vi "libera.vi"() -> ()   [LabVIEW 2012]
uses:
  chaos-common-crest/LabVIEW/LV14/chaosui-crest/chaosui-crest.lvlib
  chaos-common-crest/LabVIEW/LV14/chaosui-crest/VIs/ChaosDevState.ctl
  <vilib>/Utility/file.llb/Write To Spreadsheet File (I64).vi
  libera_env.ctl
panel:
  in  "[MT]:YYYYMMDDhhmm.ss":string
  in  "value":string
  in  "Set Environment":T1
  out "DD2":cluster{"VA":i32, "VB":i32, "VC":i32, "VD":i32}(graph)
  out "SA":cluster{"VA":i32, "VB":i32, "VC":i32, "VD":i32}(graph)
  out "DD":cluster{i32[], i32[]}[](graph)
  in  "DataFile":path
  out "libera_error":i32
  out "STATUS":string
  out "SA_OUT":T2(array[cluster])
  out "ADC_CW":T3(array[cluster])
  out "AVG_OUT":cluster{"AVG":i32}[](array[cluster])
  out "ADC_SP":T4(array[cluster])
  in  "AVG":bool=TRUE
  in  "STATE":bool=TRUE
  in  "stop":bool
  in  "loops":i32=10
  in  "DECIMATED":bool
  out "DD_OUT":T5(array[cluster])
  in  "refresh (ms)":u32=200
  out "samples":i32
  out "mode":i32
  out "Device State":T6
  out "nok":i32
  out "dev_error":bool
  out "acquisitions":u64
  out "timestamp":u64
  in  "Samples":u32=10
  in  "TRIGGERED":bool
  in  "ADC CW":bool
  in  "ADC SP":bool
  in  "SA":bool
  in  "DD":bool
  in  "!CHAOS URL":string="chaost-webui1.chaos.lnf.infn.it:8081"
  in  "LiberaID":string="LIBERA02/LIBERA_ACQUIRE0"
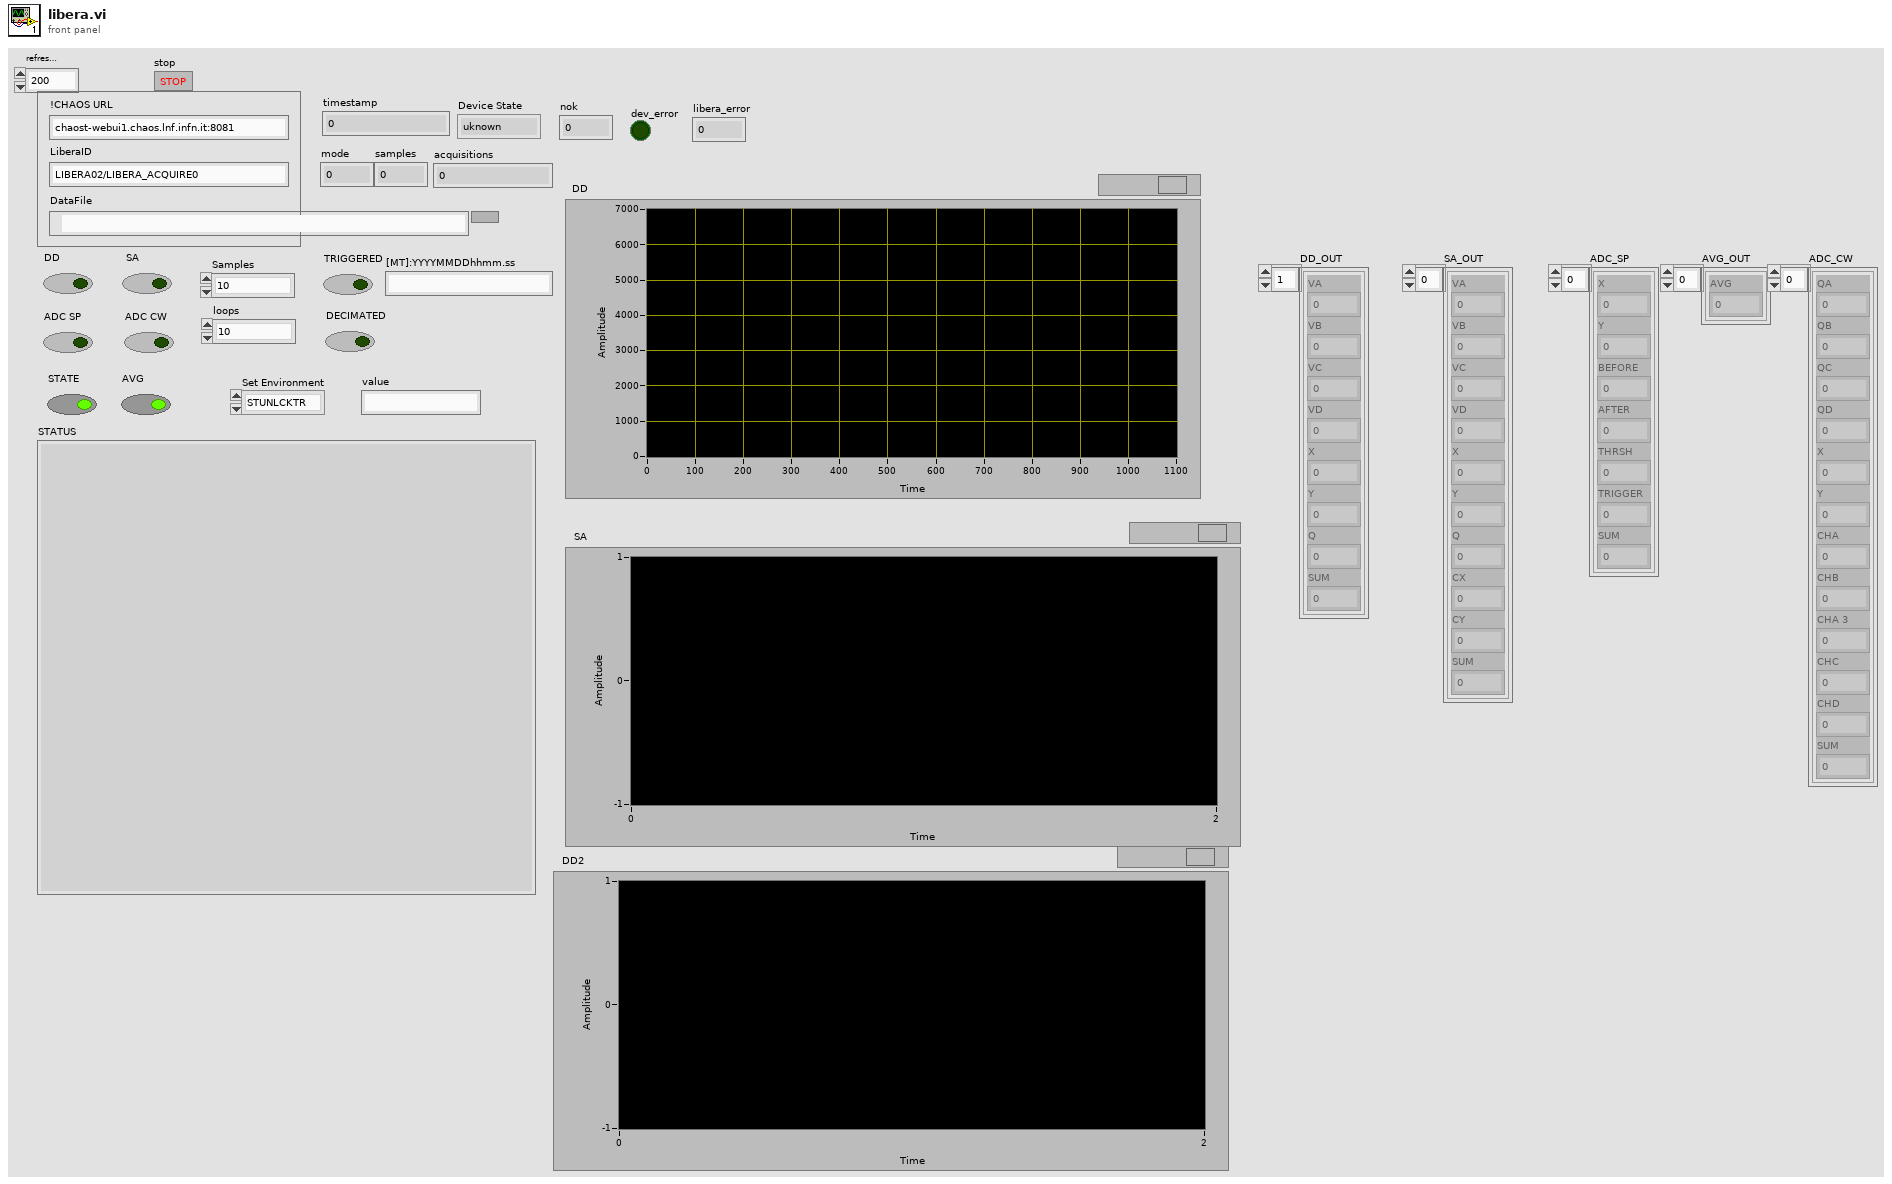
[diagram p1: front panel]
types:
  T1 = typedef "libera_env.ctl" = enum16{"STUNLCKTR", "MTSYNCIN", "MTUNLCKTR", "MTNCOSHFT", "MTVCXOFFS", "POLYPHASE_FIR", "NOTCH2", "NOTCH1", "DDC_MAFDELAY", "DDC_MAFLENGTH", "SWDELAY", "EXTSWITCH", "TRIGDELAY", "PMDEC", "PMOFFSET", "ILKSTATUS", "ILK", "DSC", "AGC", "GAIN", "SWITCH", "QOFFSET", "YOFFSET", "XOFFSET", "KY", "KX"}
  T2 = cluster{"VA":i32, "VB":i32, "VC":i32, "VD":i32, "X":i32, "Y ":i32, "Q":i32, "CX":i32, "CY":i32, "SUM":i32}[]
  T3 = cluster{"QA":i32, "QB":i32, "QC":i32, "QD":i32, "X":i32, "Y":i32, "CHA":i32, "CHB":i32, "CHA 3":i32, "CHC":i32, "CHD":i32, "SUM":i32}[]
  T4 = cluster{"X":i32, "Y":i32, "BEFORE":i32, "AFTER":i32, "THRSH":i32, "TRIGGER":i32, "SUM":i32}[]
  T5 = cluster{"VA":i32, "VB":i32, "VC":i32, "VD":i32, "X":i32, "Y ":i32, "Q":i32, "SUM":i32}[]
  T6 = typedef "ChaosDevState.ctl" = enum16{"uknown", "stop", "init", "deinit", "start"}
  T7 = typedef "LabVIEWHTTPClient.lvlib/ClientHandle.ctl" = refnum<k1>
  T8 = cluster{"client handle out":T7, "chaoswanurl":string}
  T9 = enum16{"setEnv", "stopAcquire", "setTime", "acquireAVG", "acquireADCSP", "acquireADCCW", "acquireStream", "acquireDD"}
  T10 = cluster{"VA":i32, "VB":i32, "VC":i32, "VD":i32, "X":i32, "Y ":i32, "Q":i32, "CX":i32, "CY":i32, "SUM":i32}
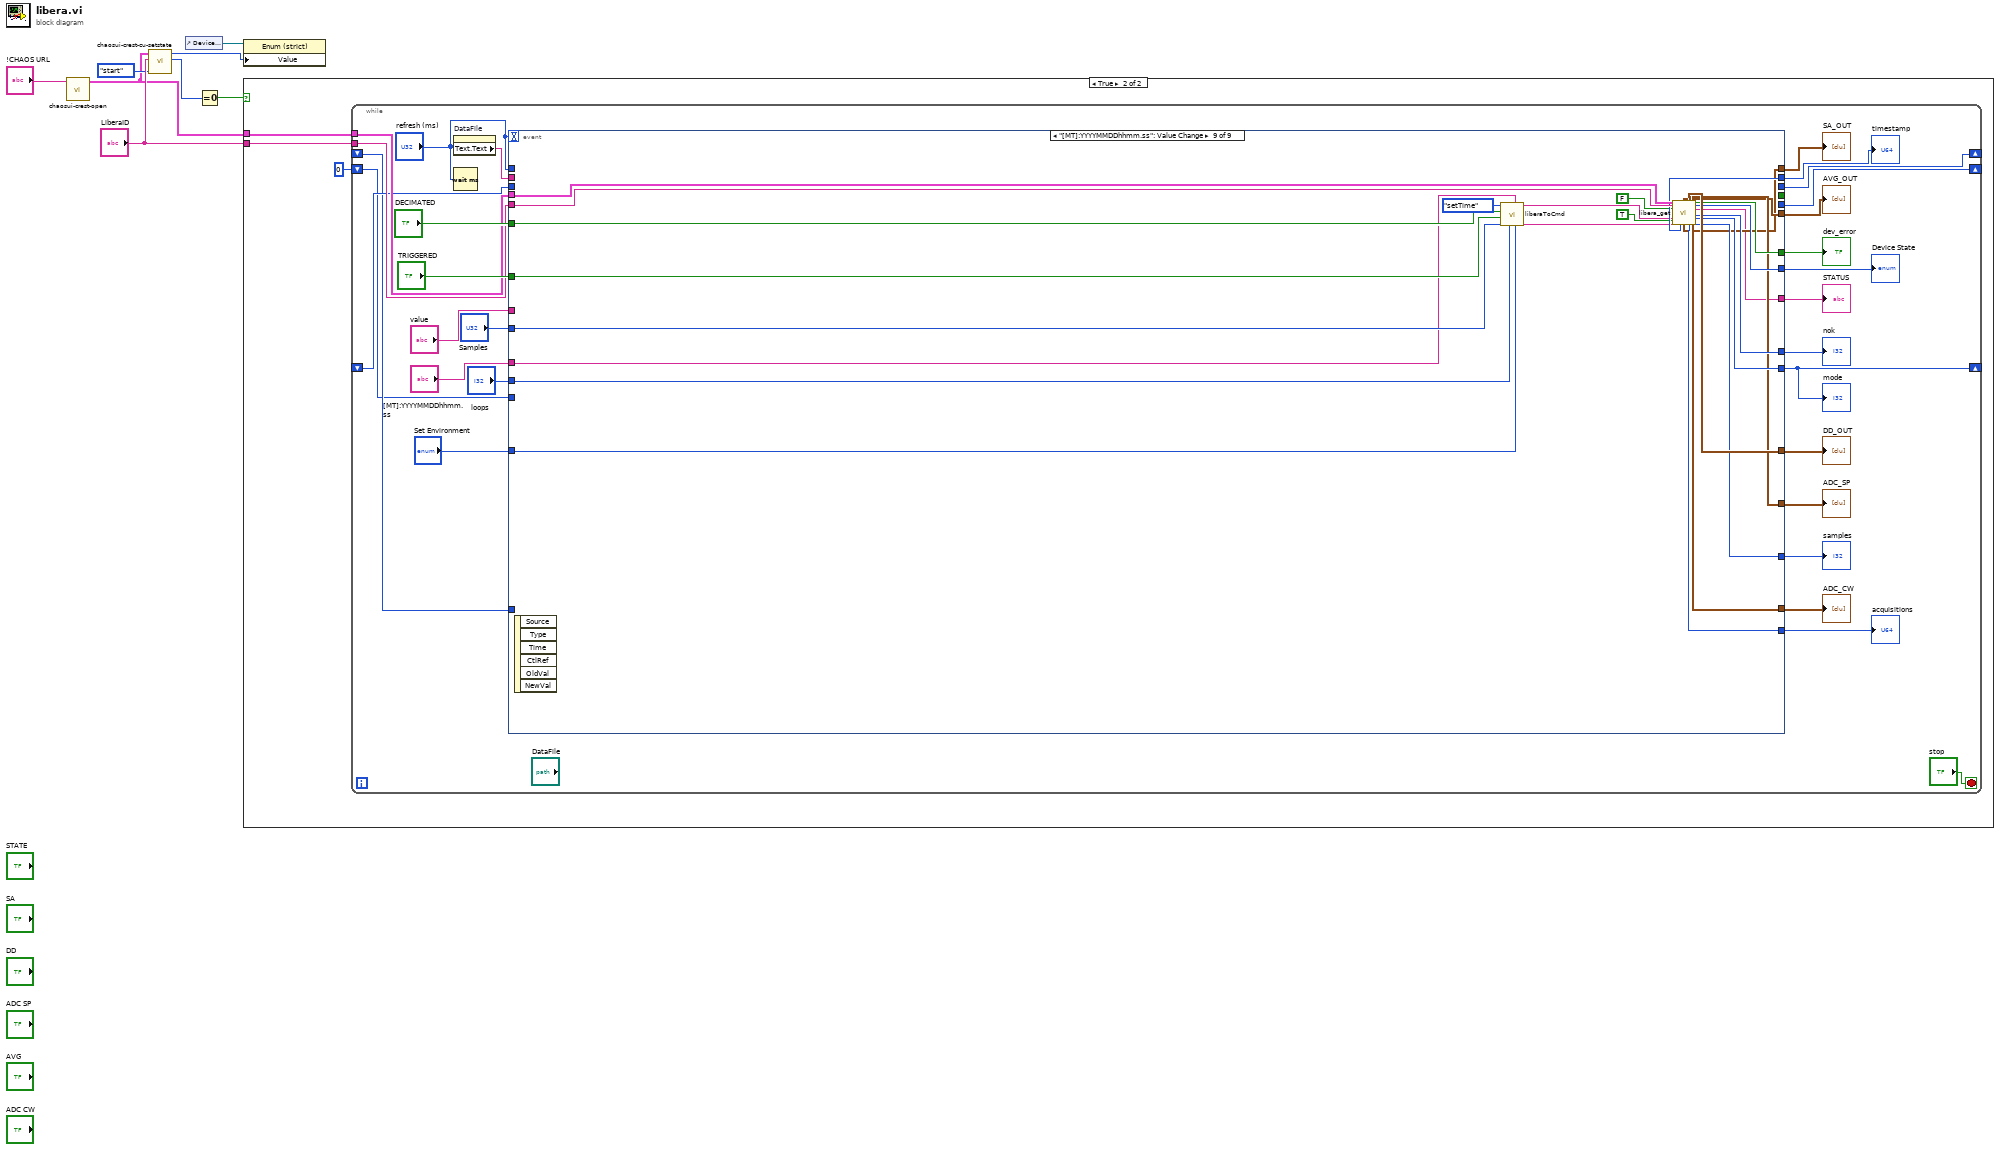
[diagram p0: block diagram]
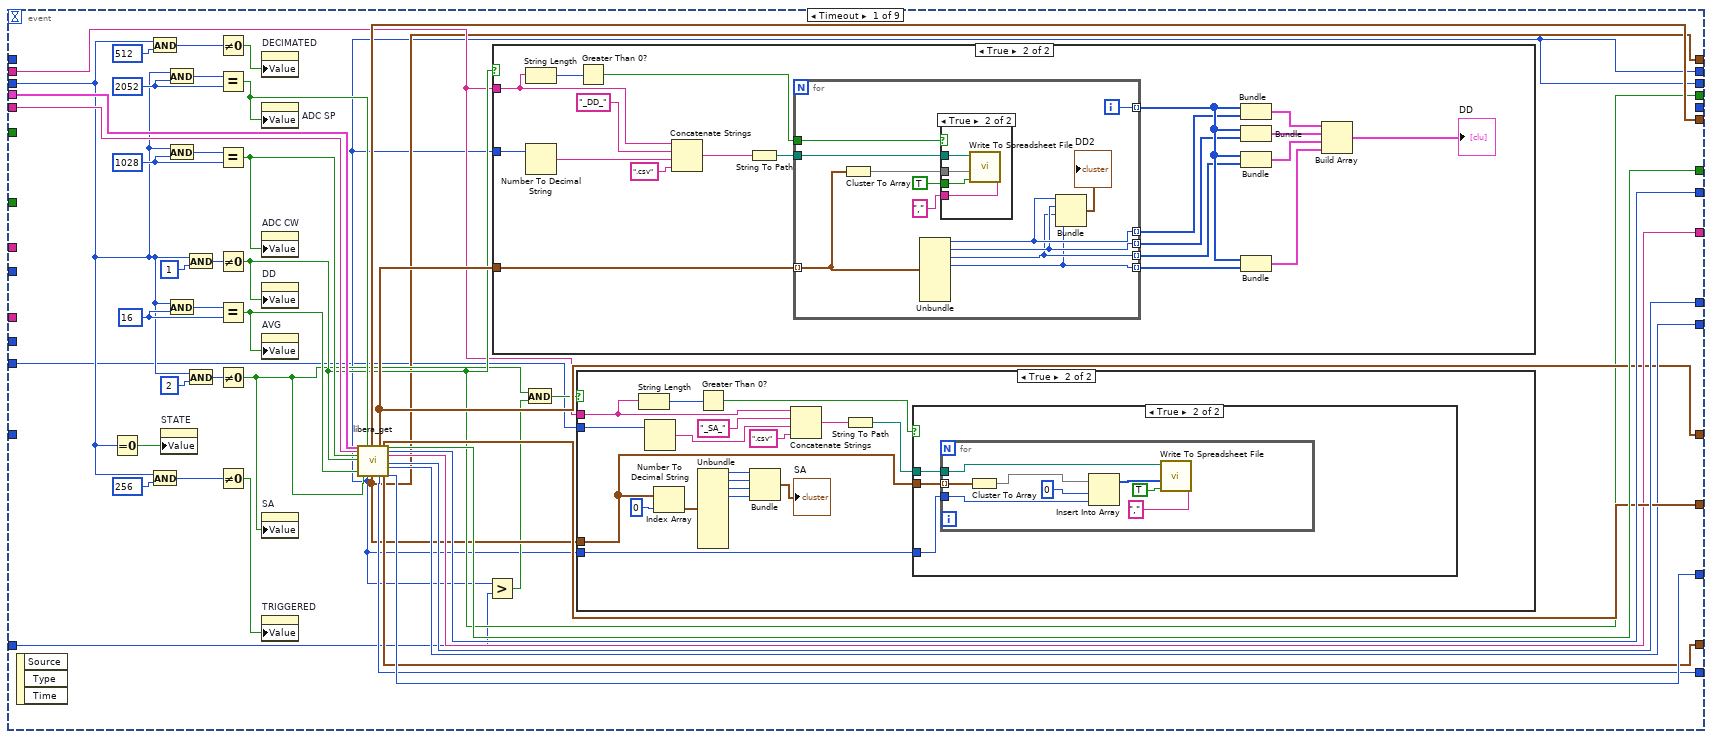
[diagram p3: hidden frame]
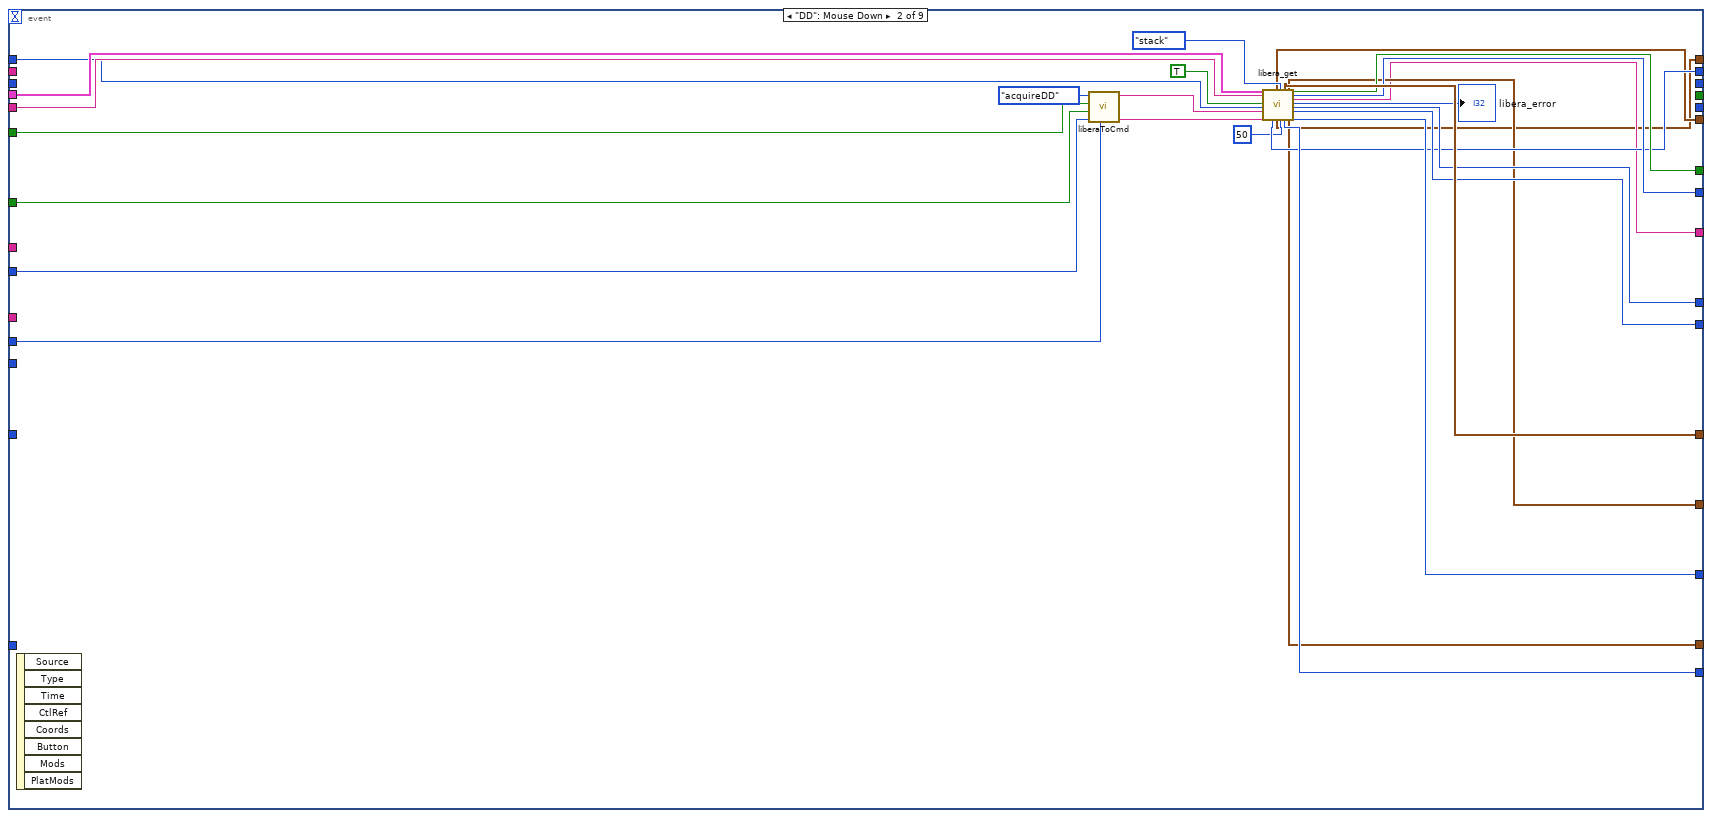
[diagram p8: hidden frame]
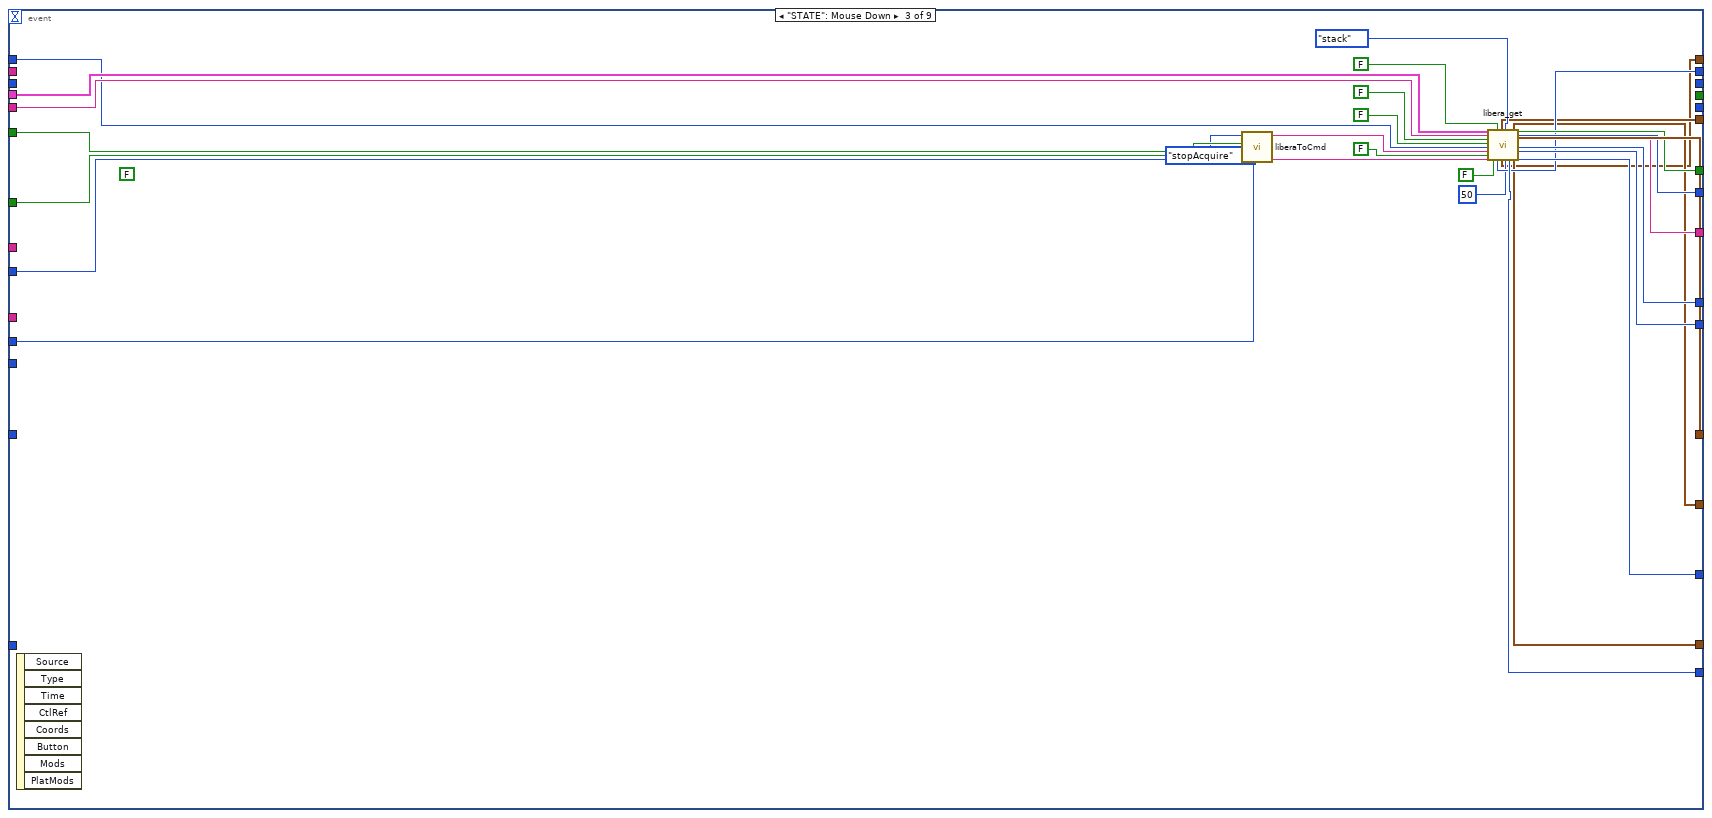
[diagram p9: hidden frame]
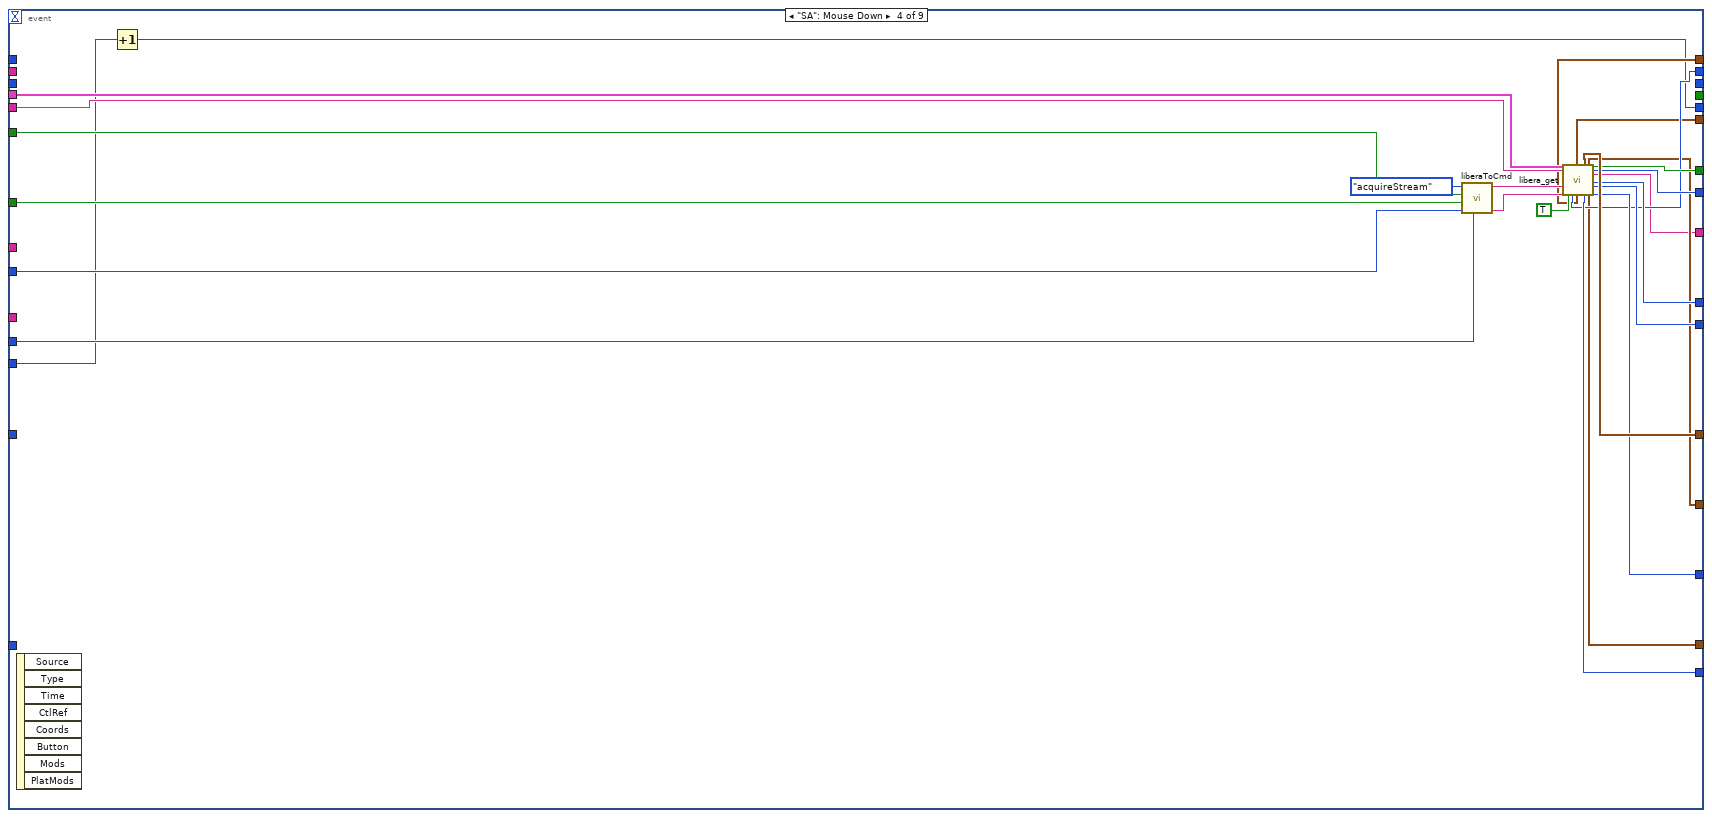
[diagram p10: hidden frame]
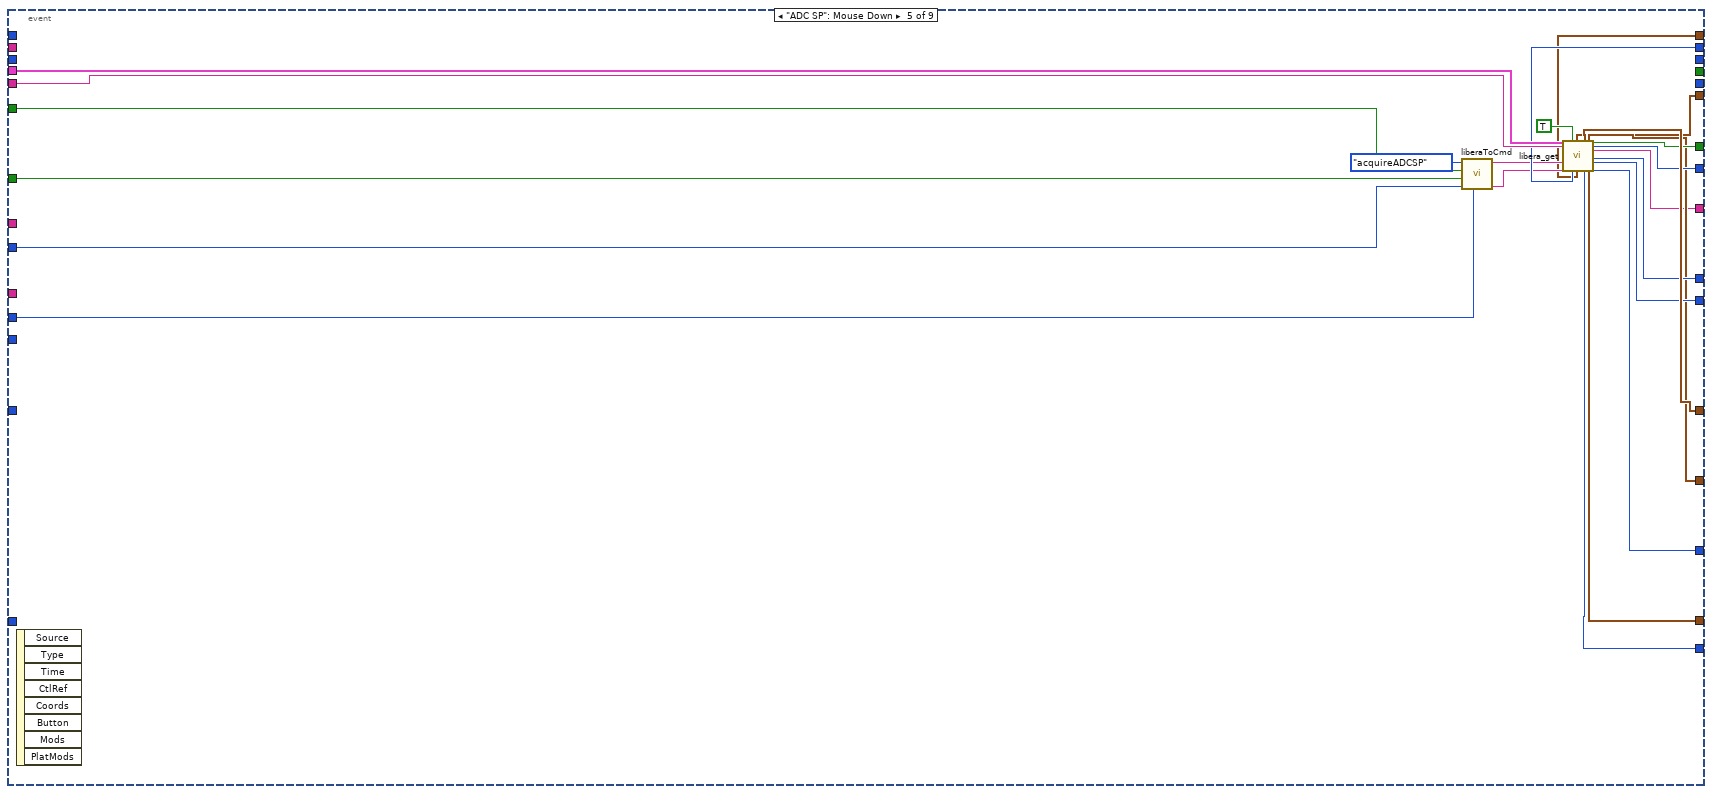
[diagram p11: hidden frame]
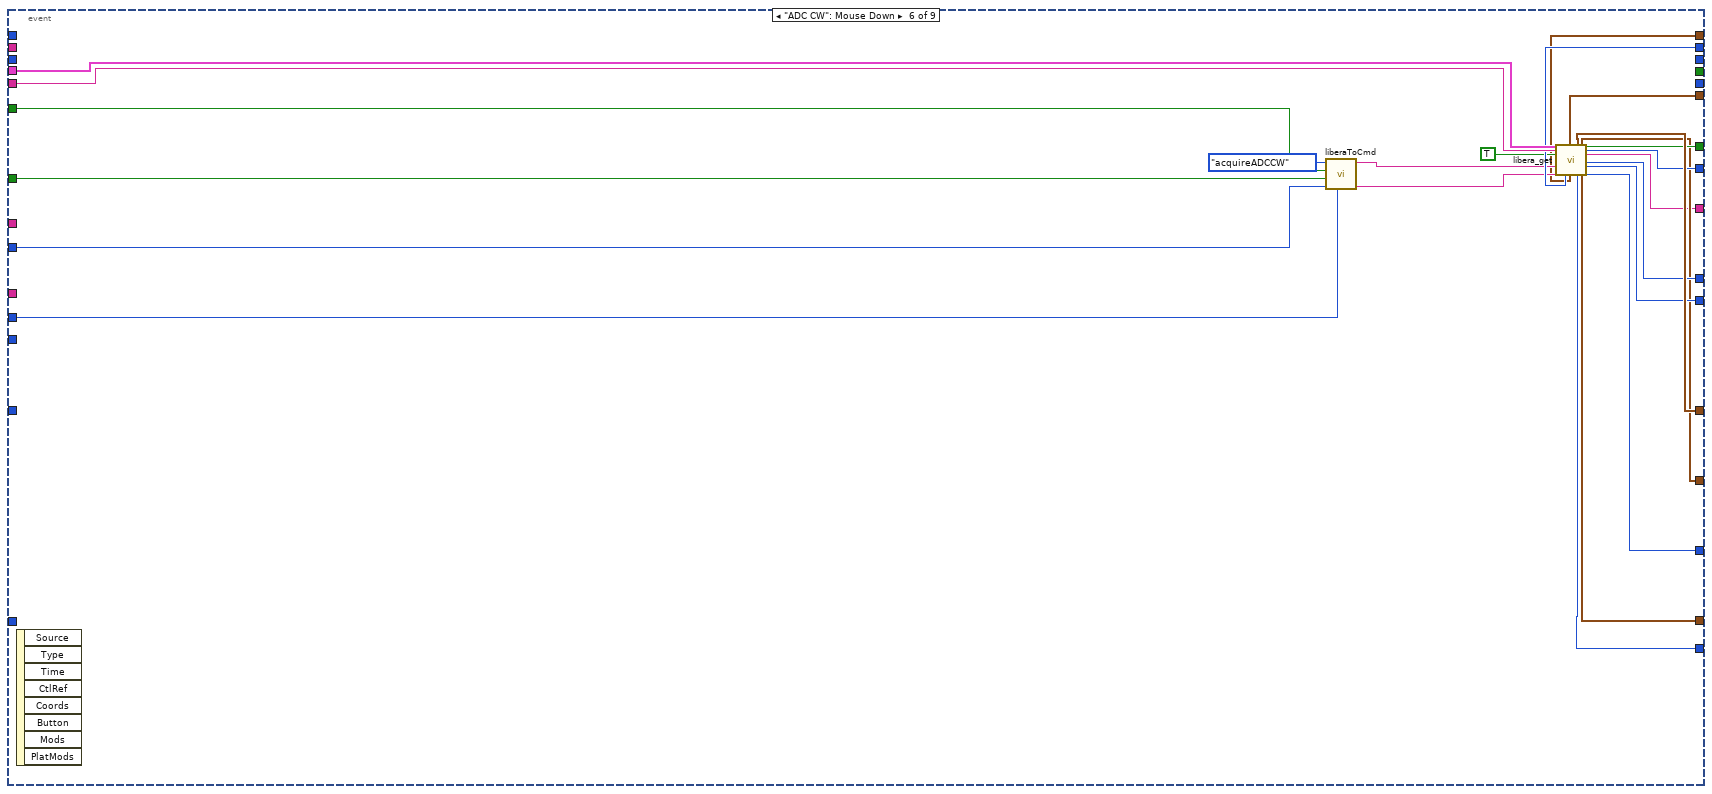
[diagram p12: hidden frame]
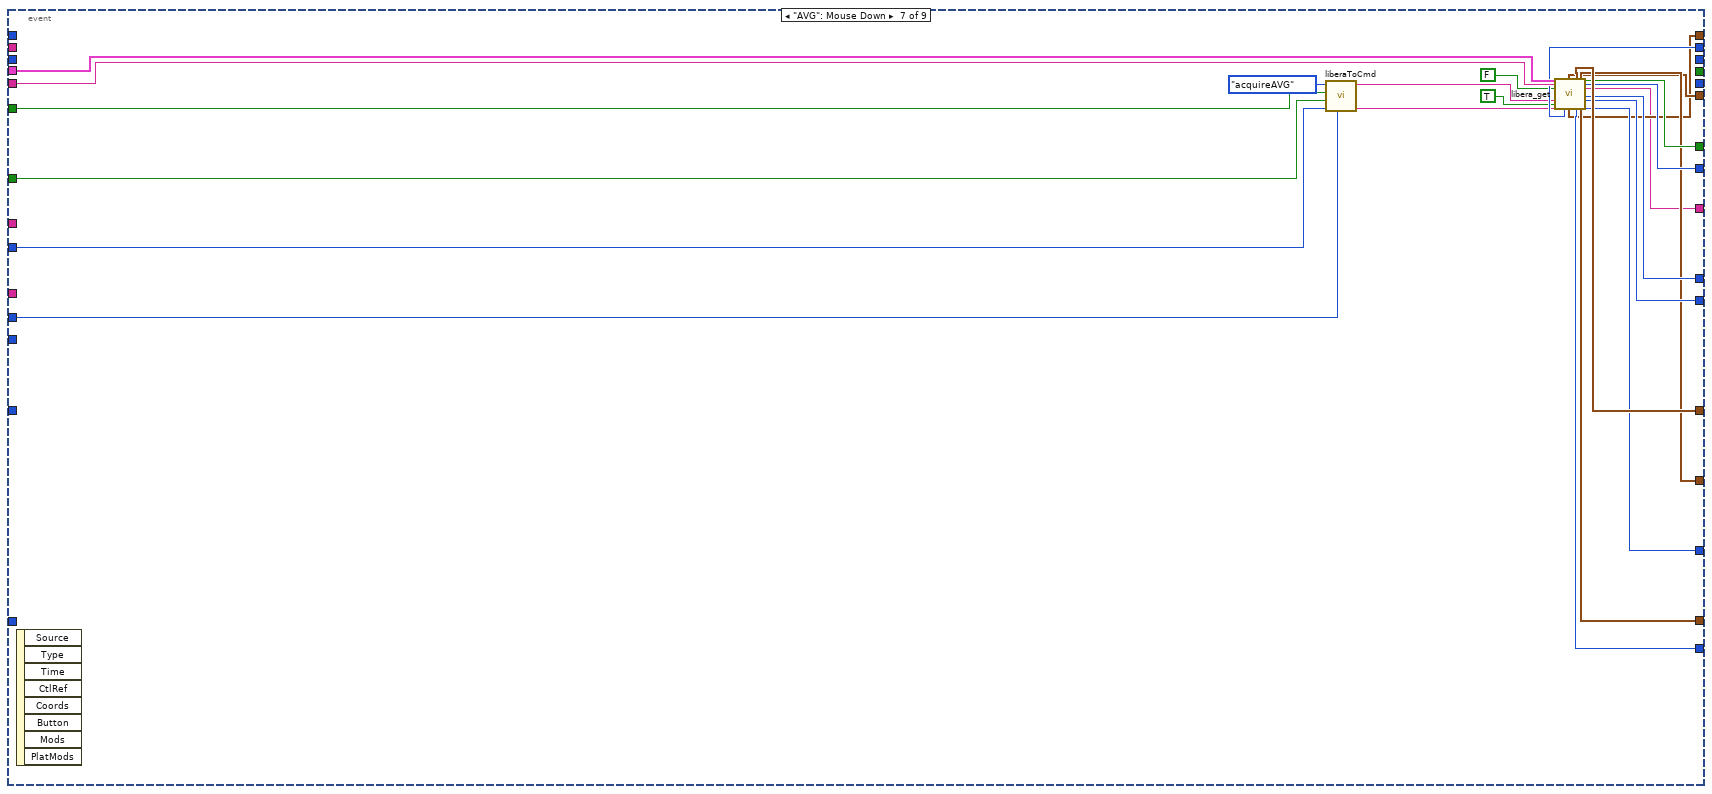
[diagram p13: hidden frame]
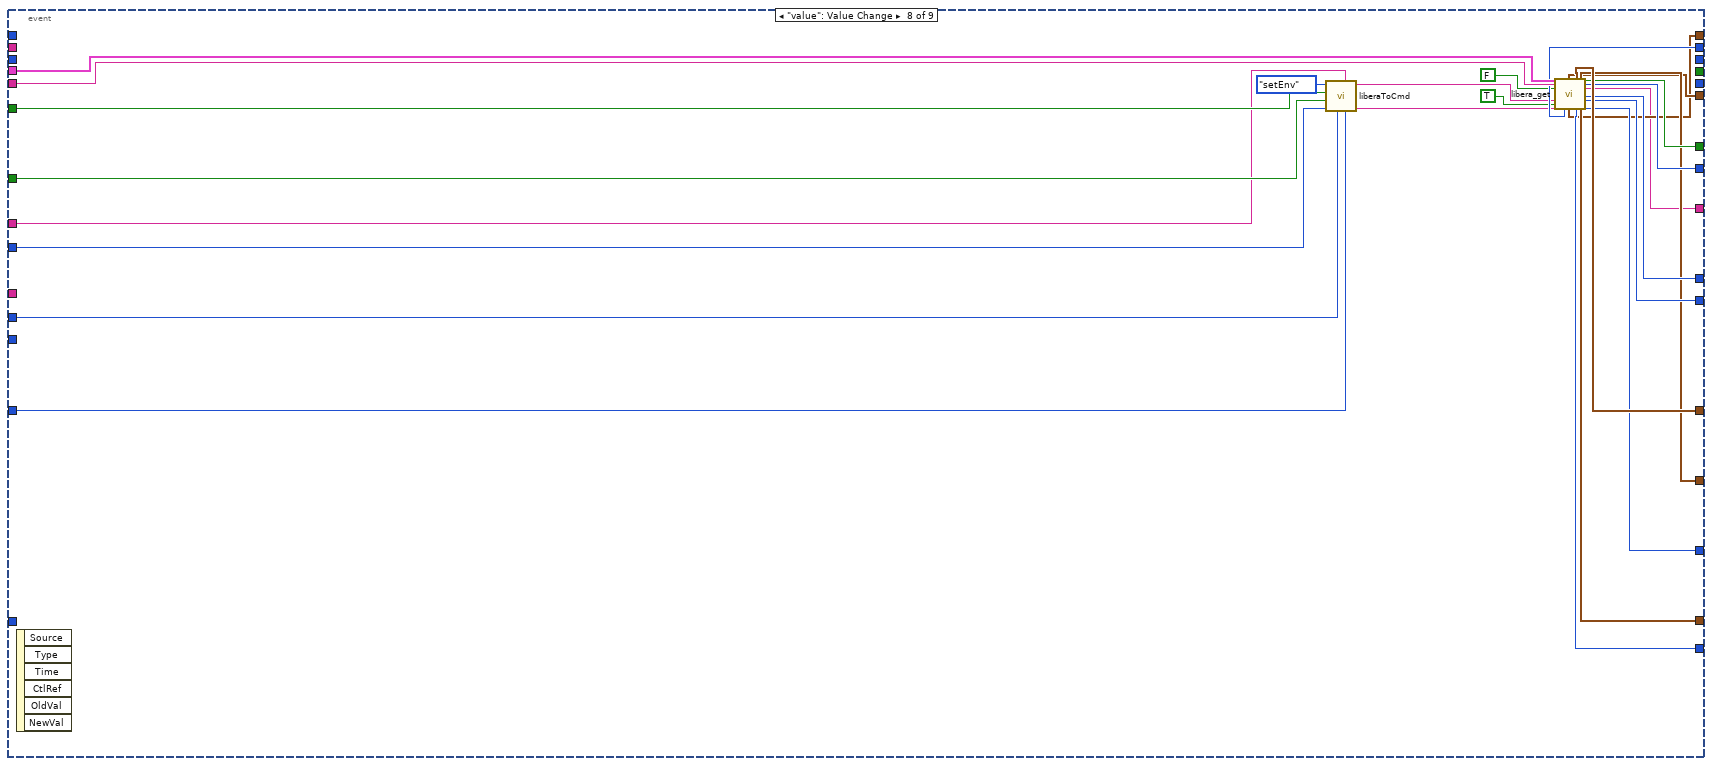
[diagram p14: hidden frame]
diagram:
  n1 = call "chaosui-crest-open.vi"("chaoswanurl"="!CHAOS URL") -> ("handle"=w1:T8)  [unwired: 10 in]
  n2 = call "chaosui-crest-cu-setstate.vi"("dev_state"=ChaosDevState."start", "cuname"="LiberaID", "handleConnection"=w1) -> ("nok"=w3:i32, "dev_state_out"=w4:T6)  [unwired: 1 in, 3 out]
  n3 = control-ref of="Device State"() -> (w5:refnum<vi>)
  n4 = Equal To 0?(x=w3) -> (x = 0?=w7:bool)
  n5 = property class="Enum (strict)"(reference=w5, "Value"=w4) -> ()  [unwired: 1 in, 2 out]
  n6 = case shown="True" w7 {
    tunnel: w1 -> [_ w11]
    tunnel: "LiberaID" -> [_ w10]
    frame False {
    }
    frame True {
      n7 = while {
        tunnel: w11 -> [w30]
        tunnel: w10 -> [w29]
        shift-right: [w28] -> _
        shift-left: _ -> [w27]
        shift-right: [w18] -> _
        shift-left: _ -> [w17]
        shift-right: [w15] -> _
        shift-left: 0 -> [w16]
        stop <- "stop" stop-if-true
        n8 = property on="DataFile" class="Path"() -> ("Text.Text"=w19:string)  [unwired: 2 in, 2 out]
        n9 = Wait (ms)(milliseconds to wait="refresh (ms)") -> ()  [unwired: 1 out]
        n10 = event shown="[8] \"[MT]:YYYYMMDDhhmm.ss\": Value Change" {
          selector: _ -> [_ _ _ _ _ _ _ _ _]
          dyn-events: _ -> [_ _ _ _ _ _ _ _ _]
          timeout: "refresh (ms)" -> [_ _ _ _ _ _ _ _ _]
          tunnel: w30 -> [w84 w176 w206 w231 w254 w277 w301 w327 w353]
          tunnel: w29 -> [w83 w175 w205 w230 w253 w276 w300 w326 w352]
          tunnel: [w82 w173 w203 w228 w251 w274 w298 w324 w350] -> w41
          tunnel: [w81 w172 w202 w227 w250 w273 w297 w323 w349] -> w40
          tunnel: [w80 w171 w201 w226 w249 w272 w296 w322 w348] -> w39
          tunnel: [w52 w170 w200 w225 w248 w271 w295 w321 w347] -> w28
          tunnel: [w79 w169 w199 w224 w247 w270 w294 w320 w346] -> w38
          tunnel: [w78 w168 w198 w223 w246 w269 w293 w319 w345] -> w37
          tunnel: [w43 w167 w197 w222 w245 w268 w292 w318 w344] -> w20
          tunnel: [w51 w174 w204 w229 w252 w275 w299 w325 w351] -> w21
          tunnel: "Samples" -> [_ w166 w196 w221 w244 w267 w291 w317 w343]
          tunnel: "TRIGGERED" -> [_ w165 w195 w220 w243 w266 w290 w316 w342]
          tunnel: "DECIMATED" -> [_ w164 w194 w219 w242 w265 w289 w315 w341]
          tunnel: "loops" -> [_ w161 w191 w216 w239 w262 w286 w312 w338]
          tunnel: "refresh (ms)" -> [_ w159 w189 _ _ _ _ _ _]
          tunnel: w27 -> [w58 _ _ _ _ _ _ _ _]
          tunnel: [w55 w156 w181 w214 w237 w260 w283 w309 w335] -> w26
          tunnel: [w53 w155 w180 w213 w236 w259 w282 w308 w334] -> w25
          tunnel: [w56 w153 w179 w210 w234 w257 w281 w307 w333] -> w24
          tunnel: [w47 w152 w178 w211 w233 w256 w280 w306 w332] -> w23
          tunnel: [w54 w154 w182 w212 w235 w258 w279 w305 w331] -> w22
          tunnel: [w50 _ _ _ _ _ _ _ _] -> _
          tunnel: w19 -> [w49 _ _ _ _ _ _ _ _]
          tunnel: [w43 _ _ _ _ _ _ _ _] -> w18
          tunnel: w17 -> [w46 _ _ _ _ _ _ _ _]
          tunnel: w16 -> [w42 _ _ w209 _ _ _ _ _]
          tunnel: [_ _ _ w208 _ _ _ _ _] -> w15
          tunnel: "Set Environment" -> [_ _ _ _ _ _ _ w303 w329]
          tunnel: "value" -> [_ _ _ _ _ _ _ w302 _]
          tunnel: "[MT]:YYYYMMDDhhmm.ss" -> [_ _ _ _ _ _ _ _ w328]
          event Timeout {
            w65 = u32 16 ("y")
            w69 = u32 1028 ("y")
            w71 = u32 2052 ("y")
            n11 = event-data() -> ()  [unwired: 1 in, 3 out]
            n12 = Equal To 0?(x=w58) -> (x = 0?=w75:bool)
            n13 = And(x=w58, y=u32 512) -> (x .and. y?=w59:u32)
            n14 = And(x=w58, y=u32 256) -> (x .and. y?=w63:u32)
            n15 = property on="STATE" class="Bool (strict)"("Value"=w75) -> ()  [unwired: 2 in, 2 out]
            n16 = And(x=w58, y=w71) -> (x .and. y?=w72:u32)
            n17 = And(x=w58, y=w69) -> (x .and. y?=w68:u32)
            n18 = And(x=w58, y=w65) -> (x .and. y?=w66:u32)
            n19 = And(x=w58, y=u32 1) -> (x .and. y?=w76:u32)
            n20 = And(x=w58, y=u32 2) -> (x .and. y?=w73:u32)
            n21 = Not Equal To 0?(x=w59) -> (x != 0?=w57:bool)
            n22 = Equal?(x=w72, y=w71) -> (x = y?=w70:bool)
            n23 = Equal?(x=w68, y=w69) -> (x = y?=w67:bool)
            n24 = Not Equal To 0?(x=w76) -> (x != 0?=w50:bool)
            n25 = Equal?(x=w66, y=w65) -> (x = y?=w64:bool)
            n26 = Not Equal To 0?(x=w73) -> (x != 0?=w48:bool)
            n27 = Not Equal To 0?(x=w63) -> (x != 0?=w61:bool)
            n28 = property on="DECIMATED" class="Bool (strict)"("Value"=w57) -> ()  [unwired: 2 in, 2 out]
            n29 = property on="ADC SP" class="Bool (strict)"("Value"=w70) -> ()  [unwired: 2 in, 2 out]
            n30 = property on="ADC CW" class="Bool (strict)"("Value"=w67) -> ()  [unwired: 2 in, 2 out]
            n31 = property on="DD" class="Bool (strict)"("Value"=w50) -> ()  [unwired: 2 in, 2 out]
            n32 = property on="AVG" class="Bool (strict)"("Value"=w64) -> ()  [unwired: 2 in, 2 out]
            n33 = property on="SA" class="Bool (strict)"("Value"=w48) -> ()  [unwired: 2 in, 2 out]
            n34 = property on="TRIGGERED" class="Bool (strict)"("Value"=w61) -> ()  [unwired: 2 in, 2 out]
            n35 = call "libera_get.vi"("handleConnection"=w84, "cuname"=w83, "Enable ADC CW"=w67, "Enable DD"=w50, "Enable AVG"=w64, "Enable SA"=w48, "Enable ADC SP"=w70) -> ("timestamp"=w43:u64, "AVG"=w53:cluster{"AVG":i32}[], "SA"=w47:T2, "DD"=w51:T5, "acquisitions"=w78:u64, "ADC_SP"=w55:T4, "ADC_CW"=w56:T3, "dev_error"=w82:bool, "dev_state"=w81:T6, "STATUS"=w54:string, "nok"=w80:i32, "mode"=w52:i32, "samples"=w79:i32)  [unwired: 7 in, 1 out]
            n36 = Greater?(x=w43, y=w46) -> (0:w44:bool)
            n37 = case shown="True" w50 {
              tunnel: w43 -> [_ w133]
              tunnel: w51 -> [_ w127]
              tunnel: w49 -> [_ w119]
              frame False {
              }
              frame True {
                n38 = String Length(string=w119) -> (length=w120:i32)
                n39 = Number To Decimal String(number=w133) -> (decimal integer string=w132:string)  [unwired: 1 in]
                n40 = Greater Than 0?(x=w120) -> (x > 0?=w118:bool)
                n41 = Concatenate Strings(w119, "_DD_" ("string"), w132, ".csv" ("name or relative path")) -> (w129:string)
                n42 = String To Path(string=w129) -> (path=w128:path)
                n43 = for {
                  tunnel: w128 -> [w145]
                  tunnel: w127 -> [w141] mode=indexing
                  tunnel: [w138] -> w114 mode=indexing
                  tunnel: [w140] -> w126 mode=indexing
                  tunnel: [w137] -> w117 mode=indexing
                  tunnel: [w136] -> w116 mode=indexing
                  tunnel: [w135] -> w115 mode=indexing
                  tunnel: w118 -> [w139]
                  i -> [w140]
                  n44 = Cluster To Array(cluster=w141) -> (array=w144:i32[])
                  n45 = Unbundle(w141) -> ("VA"=w138:i32, "VB"=w137:i32, "VC"=w136:i32, "VD"=w135:i32)  [unwired: 4 out]
                  n46 = case shown="True" w139 {
                    tunnel: w145 -> [_ w149]
                    tunnel: w144 -> [_ w148]
                    tunnel: TRUE ("append to file? (new file:F)") -> [_ w147]
                    tunnel: "," ("delimiter (\\t)") -> [_ w146]
                    frame False {
                    }
                    frame True {
                      n47 = call-poly <vilib>:"Write To Spreadsheet File.vi"("delimiter (\\t)"=w146, "append to file? (new file:F)"=w147, "1D data"=w148, "file path (dialog if empty)"=w149) -> ()  [unwired: 4 in, 1 out]
                    }
                  }
                  n48 = Bundle("VA"=w138, "VB"=w137, "VC"=w136, "VD"=w135) -> (→"DD2":cluster{"VA":i32, "VB":i32, "VC":i32, "VD":i32})  [unwired: 1 in]
                }
                n49 = Bundle(w126, w114) -> (w125:cluster{i32[], i32[]})  [unwired: 1 in]
                n50 = Bundle(w126, w117) -> (w124:cluster{i32[], i32[]})  [unwired: 1 in]
                n51 = Bundle(w126, w116) -> (w123:cluster{i32[], i32[]})  [unwired: 1 in]
                n52 = Bundle(w126, w115) -> (w122:cluster{i32[], i32[]})  [unwired: 1 in]
                n53 = Build Array(w125, w124, w123, w122) -> (→"DD":cluster{i32[], i32[]}[])
              }
            }
            n54 = And(x=w48, y=w44) -> (x .and. y?=w45:bool)
            n55 = case shown="True" w45 {
              tunnel: w47 -> [_ w97]
              tunnel: w49 -> [_ w90]
              tunnel: w43 -> [_ w94]
              tunnel: w42 -> [_ w99]
              frame False {
              }
              frame True {
                n56 = String Length(string=w90) -> (length=w91:i32)
                n57 = Number To Decimal String(number=w99) -> (decimal integer string=w98:string)  [unwired: 1 in]
                n58 = Index Array(array=w97, index=0) -> (element=w95:T10)
                n59 = Greater Than 0?(x=w91) -> (x > 0?=w92:bool)
                n60 = Unbundle(w95) -> ("VA"=w89:i32, "VB"=w88:i32, "VC"=w87:i32, "VD"=w86:i32)  [unwired: 6 out]
                n61 = Bundle("VA"=w89, "VB"=w88, "VC"=w87, "VD"=w86) -> (→"SA":cluster{"VA":i32, "VB":i32, "VC":i32, "VD":i32})  [unwired: 1 in]
                n62 = Concatenate Strings(w90, "_SA_" ("string"), w98, ".csv" ("name or relative path")) -> (w101:string)
                n63 = String To Path(string=w101) -> (path=w100:path)
                n64 = case shown="True" w92 {
                  tunnel: w100 -> [_ w105]
                  tunnel: w97 -> [_ w104]
                  tunnel: w94 -> [_ w103]
                  frame False {
                  }
                  frame True {
                    n65 = for {
                      tunnel: w105 -> [w113]
                      tunnel: w104 -> [w112] mode=indexing
                      tunnel: w103 -> [w107]
                      n66 = Cluster To Array(cluster=w112) -> (array=w109:i32[])
                      n67 = Insert Into Array(array=w109, index=0, new element=w107) -> (w106:i32[])
                      n68 = call-poly <vilib>:"Write To Spreadsheet File.vi"("delimiter (\\t)"="," ("delimiter (\\t)"), "append to file? (new file:F)"=TRUE, "1D data"=w106, "file path (dialog if empty)"=w113) -> ()  [unwired: 4 in, 1 out]
                    }
                  }
                }
              }
            }
          }
          event "DD": Mouse Down {
            n69 = event-data() -> ()  [unwired: 1 in, 8 out]
            n70 = call "liberaToCmd.vi"("loops"=w161, "samples"=w166, "triggered"=w165, "decimated"=w164, "cmd"=T9."acquireDD") -> ("jsonargs"=w162:string, "cmd"=w163:string)  [unwired: 5 in]
            n71 = call "libera_get.vi"("handleConnection"=w176, "cuname"=w175, "Enable DD"=TRUE, "sched (ms)"=w159, "cmd"=w163, "args"=w162, "cmd submission mode"=enum16{"stack", "kill previous"}."stack", "prio"=50) -> ("timestamp"=w167:u64, "AVG"=w155:cluster{"AVG":i32}[], "SA"=w152:T2, "DD"=w174:T5, "acquisitions"=w168:u64, "ADC_SP"=w156:T4, "ADC_CW"=w153:T3, "dev_error"=w173:bool, "dev_state"=w172:T6, "STATUS"=w154:string, "libera_error"=→"libera_error":i32, "nok"=w171:i32, "mode"=w170:i32, "samples"=w169:i32)  [unwired: 6 in]
          }
          event "STATE": Mouse Down {
            (unwired) FALSE ("Enable SA")
            n72 = event-data() -> ()  [unwired: 1 in, 8 out]
            n73 = call "liberaToCmd.vi"("loops"=w191, "samples"=w196, "triggered"=w195, "decimated"=w194, "cmd"=T9."stopAcquire") -> ("jsonargs"=w192:string, "cmd"=w193:string)  [unwired: 5 in]
            n74 = call "libera_get.vi"("handleConnection"=w206, "cuname"=w205, "Enable ADC CW"=FALSE, "Enable DD"=FALSE, "sched (ms)"=w189, "cmd"=w193, "Enable AVG"=FALSE, "args"=w192, "Enable SA"=FALSE, "Enable ADC SP"=FALSE, "cmd submission mode"=enum16{"stack", "kill previous"}."stack", "prio"=50) -> ("timestamp"=w197:u64, "AVG"=w180:cluster{"AVG":i32}[], "SA"=w178:T2, "DD"=w204:T5, "acquisitions"=w198:u64, "ADC_SP"=w181:T4, "ADC_CW"=w179:T3, "dev_error"=w203:bool, "dev_state"=w202:T6, "STATUS"=w182:string, "nok"=w201:i32, "mode"=w200:i32, "samples"=w199:i32)  [unwired: 2 in, 1 out]
          }
          event "SA": Mouse Down {
            n75 = event-data() -> ()  [unwired: 1 in, 8 out]
            n76 = Increment(x=w209) -> (x+1=w208:i32)
            n77 = call "liberaToCmd.vi"("loops"=w216, "samples"=w221, "triggered"=w220, "decimated"=w219, "cmd"=T9."acquireStream") -> ("jsonargs"=w217:string, "cmd"=w218:string)  [unwired: 5 in]
            n78 = call "libera_get.vi"("handleConnection"=w231, "cuname"=w230, "cmd"=w218, "args"=w217, "Enable SA"=TRUE) -> ("timestamp"=w222:u64, "AVG"=w213:cluster{"AVG":i32}[], "SA"=w211:T2, "DD"=w229:T5, "acquisitions"=w223:u64, "ADC_SP"=w214:T4, "ADC_CW"=w210:T3, "dev_error"=w228:bool, "dev_state"=w227:T6, "STATUS"=w212:string, "nok"=w226:i32, "mode"=w225:i32, "samples"=w224:i32)  [unwired: 9 in, 1 out]
          }
          event "ADC SP": Mouse Down {
            n79 = event-data() -> ()  [unwired: 1 in, 8 out]
            n80 = call "liberaToCmd.vi"("loops"=w239, "samples"=w244, "triggered"=w243, "decimated"=w242, "cmd"=T9."acquireADCSP") -> ("jsonargs"=w240:string, "cmd"=w241:string)  [unwired: 5 in]
            n81 = call "libera_get.vi"("handleConnection"=w254, "cuname"=w253, "cmd"=w241, "args"=w240, "Enable ADC SP"=TRUE) -> ("timestamp"=w245:u64, "AVG"=w236:cluster{"AVG":i32}[], "SA"=w233:T2, "DD"=w252:T5, "acquisitions"=w246:u64, "ADC_SP"=w237:T4, "ADC_CW"=w234:T3, "dev_error"=w251:bool, "dev_state"=w250:T6, "STATUS"=w235:string, "nok"=w249:i32, "mode"=w248:i32, "samples"=w247:i32)  [unwired: 9 in, 1 out]
          }
          event "ADC CW": Mouse Down {
            n82 = event-data() -> ()  [unwired: 1 in, 8 out]
            n83 = call "liberaToCmd.vi"("loops"=w262, "samples"=w267, "triggered"=w266, "decimated"=w265, "cmd"=T9."acquireADCCW") -> ("jsonargs"=w263:string, "cmd"=w264:string)  [unwired: 5 in]
            n84 = call "libera_get.vi"("handleConnection"=w277, "cuname"=w276, "Enable ADC CW"=TRUE, "cmd"=w264, "args"=w263) -> ("timestamp"=w268:u64, "AVG"=w259:cluster{"AVG":i32}[], "SA"=w256:T2, "DD"=w275:T5, "acquisitions"=w269:u64, "ADC_SP"=w260:T4, "ADC_CW"=w257:T3, "dev_error"=w274:bool, "dev_state"=w273:T6, "STATUS"=w258:string, "nok"=w272:i32, "mode"=w271:i32, "samples"=w270:i32)  [unwired: 9 in, 1 out]
          }
          event "AVG": Mouse Down {
            n85 = event-data() -> ()  [unwired: 1 in, 8 out]
            n86 = call "liberaToCmd.vi"("loops"=w286, "samples"=w291, "triggered"=w290, "decimated"=w289, "cmd"=T9."acquireAVG") -> ("jsonargs"=w287:string, "cmd"=w288:string)  [unwired: 5 in]
            n87 = call "libera_get.vi"("handleConnection"=w301, "cuname"=w300, "Enable ADC CW"=FALSE, "cmd"=w288, "Enable AVG"=TRUE, "args"=w287) -> ("timestamp"=w292:u64, "AVG"=w282:cluster{"AVG":i32}[], "SA"=w280:T2, "DD"=w299:T5, "acquisitions"=w293:u64, "ADC_SP"=w283:T4, "ADC_CW"=w281:T3, "dev_error"=w298:bool, "dev_state"=w297:T6, "STATUS"=w279:string, "nok"=w296:i32, "mode"=w295:i32, "samples"=w294:i32)  [unwired: 8 in, 1 out]
          }
          event "value": Value Change {
            n88 = event-data() -> ()  [unwired: 1 in, 6 out]
            n89 = call "liberaToCmd.vi"("Set Environment"=w303, "value"=w302, "loops"=w312, "samples"=w317, "triggered"=w316, "decimated"=w315, "cmd"=T9."setEnv") -> ("jsonargs"=w313:string, "cmd"=w314:string)  [unwired: 3 in]
            n90 = call "libera_get.vi"("handleConnection"=w327, "cuname"=w326, "Enable ADC CW"=FALSE, "cmd"=w314, "Enable AVG"=TRUE, "args"=w313) -> ("timestamp"=w318:u64, "AVG"=w308:cluster{"AVG":i32}[], "SA"=w306:T2, "DD"=w325:T5, "acquisitions"=w319:u64, "ADC_SP"=w309:T4, "ADC_CW"=w307:T3, "dev_error"=w324:bool, "dev_state"=w323:T6, "STATUS"=w305:string, "nok"=w322:i32, "mode"=w321:i32, "samples"=w320:i32)  [unwired: 8 in, 1 out]
          }
          event "[MT]:YYYYMMDDhhmm.ss": Value Change {
            n91 = event-data() -> ()  [unwired: 1 in, 6 out]
            n92 = call "liberaToCmd.vi"("Set Environment"=w329, "value"=w328, "loops"=w338, "samples"=w343, "triggered"=w342, "decimated"=w341, "cmd"=T9."setTime") -> ("jsonargs"=w339:string, "cmd"=w340:string)  [unwired: 3 in]
            n93 = call "libera_get.vi"("handleConnection"=w353, "cuname"=w352, "Enable ADC CW"=FALSE, "cmd"=w340, "Enable AVG"=TRUE, "args"=w339) -> ("timestamp"=w344:u64, "AVG"=w334:cluster{"AVG":i32}[], "SA"=w332:T2, "DD"=w351:T5, "acquisitions"=w345:u64, "ADC_SP"=w335:T4, "ADC_CW"=w333:T3, "dev_error"=w350:bool, "dev_state"=w349:T6, "STATUS"=w331:string, "nok"=w348:i32, "mode"=w347:i32, "samples"=w346:i32)  [unwired: 8 in, 1 out]
          }
        }
        "timestamp" <- w20
        "acquisitions" <- w37
        "dev_error" <- w41
        "nok" <- w39
        "Device State" <- w40
        "mode" <- w28
        "samples" <- w38
        "DD_OUT" <- w21
        "ADC_SP" <- w26
        "AVG_OUT" <- w25
        "ADC_CW" <- w24
        "SA_OUT" <- w23
        "STATUS" <- w22
      }
    }
  }
